vi "Configure Sequencer Connector.vi"(8 "error in (no error)":errorcluster, 9 "Connector (\"IF1OUT\")":string="IF1OUT", 10 "Instance (1)":i32=1, 11 "VISA resource name":refnum<visa-resource-name>) -> (0 "error out":errorcluster, 3 "VISA resource name out":refnum<visa-resource-name>)   [LabVIEW 2020, in "Rohde&Schwarz CMXP GPRF.lvlib"]
doc: "Selects the output connector for the generated signal.\n\nAttribute:\nRSCMXPGPRF_ATTR_SEQUENCER_CONNECTOR\n\nRemote-control command:\nROUTe:GPRF:GEN<i>:SPATh"
uses:
  <instrlib>/Rohde&Schwarz CMXP GPRF/Rohde&Schwarz CMXP GPRF.lvlib
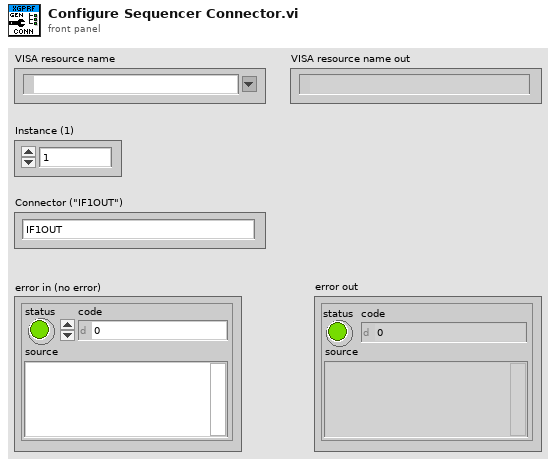
[diagram p1: front panel]
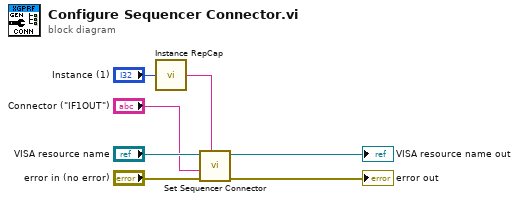
[diagram p0: block diagram]
diagram:
  n1 = call <instrlib>:"Instance RepCap.vi"("Instance in"="Instance (1)") -> ("Instance out"=w2:string)
  n2 = call "Set Sequencer Connector"("Repeated Capabilities"=w2, "error in (no error)"="error in (no error)", "Sequencer Connector ()"="Connector (\"IF1OUT\")", "instrument handle"="VISA resource name") -> ("error out"=→"error out":errorcluster, "instrument handle out"=→"VISA resource name out":refnum<visa-resource-name>)  [unwired: 6 in]
